vi "tag not found.vi"(8 "error in":errorcluster, 11 "name":string) -> (0 "error out":errorcluster)   [LabVIEW 2013, in "data bus dictionary.lvclass"]
doc: "Returns an error indicating that the tag was not found."
uses:
  data bus dictionary.lvclass
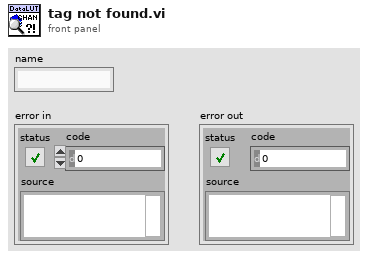
[diagram p1: front panel]
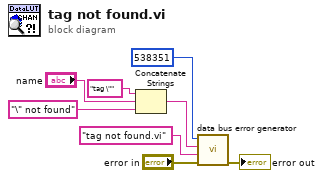
[diagram p0: block diagram]
diagram:
  n1 = Concatenate Strings("tag \"" ("format string"), "name", "\" not found" ("format string")) -> (w3:string)
  n2 = call "data bus error generator.vi"("error in"="error in", "source"="tag not found.vi", "append error message"=w3, "error code (0)"=538351) -> ("error out"=→"error out":errorcluster)  [unwired: 5 in]
